vi "3.2.0 Kalman Observation Matrix H.vi"(1 "State Vector X":T1) -> (0 "Real Matrix":T2)   [LabVIEW 2010]
uses:
  <vilib>/Analysis/Matrix/Datatypes/RealMatrix.ctl
  4-High Neurons/4.2/4.2.0 Kalman State.ctl
  <vilib>/Analysis/Matrix/Numeric/Conversions/Array To Matrix - RA2.vi
  <vilib>/Analysis/Matrix/NI_Matrix.lvlib
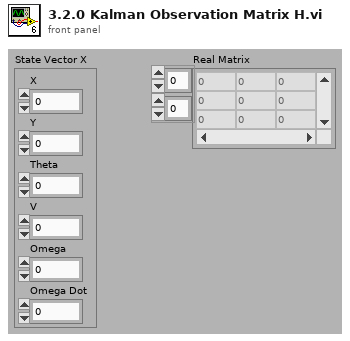
[diagram p1: front panel]
types:
  T1 = typedef "4.2.0 Kalman State.ctl" = cluster{"X":dbl, "Y":dbl, "Theta":dbl, "V":dbl, "Omega":dbl, "Omega Dot":dbl}
  T2 = typedef "NI_Matrix.lvlib/RealMatrix.ctl" = dbl[][]
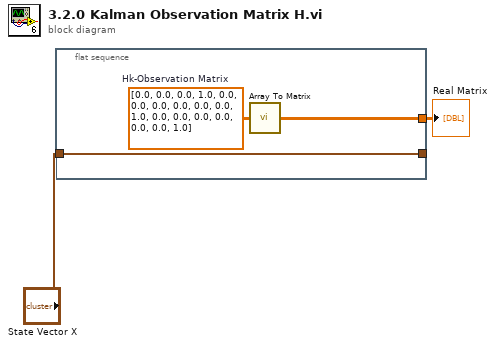
[diagram p0: block diagram]
diagram:
  n1 = flat-sequence {
    tunnel: [w4] -> _
    tunnel: "State Vector X" -> [w4]
    tunnel: [w3] -> w2
    frame #0 {
      w5 = dbl[][] [[0.0, 0.0, 0.0, 1.0, 0.0, 0.0], [0.0, 0.0, 0.0, 0.0, 1.0, 0.0], [0.0, 0.0, 0.0, 0.0, 0.0, 1.0]]  # Hk-Observation Matrix
      n2 = call-poly <vilib>:"Array To Matrix.vi"("Real 2D Array"=w5) -> ("Real Matrix"=w3:T2)
    }
  }
  "Real Matrix" <- w2
